vi "Query.vi"(6 "delay (55ms)":u32=55, 8 "error in (no error)":errorcluster, 10 "data in":string, 11 "refnum in":refnum<visa-resource-name>) -> (0 "error out":errorcluster, 2 "data out":string, 3 "refnum out":refnum<visa-resource-name>)   [LabVIEW 2020, in "Korad KA3305P.lvlib"]
uses:
  Korad KA3305P.lvlib
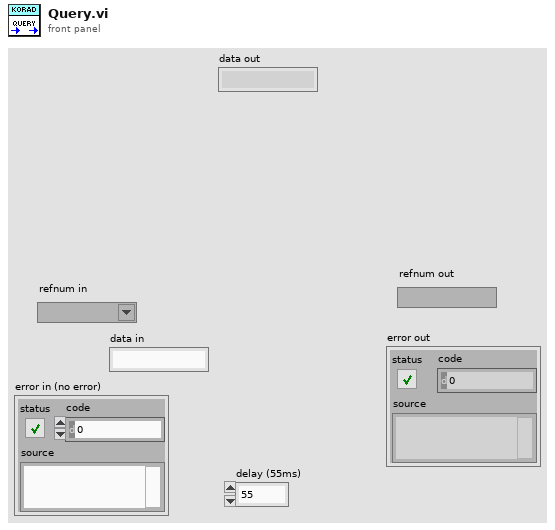
[diagram p1: front panel]
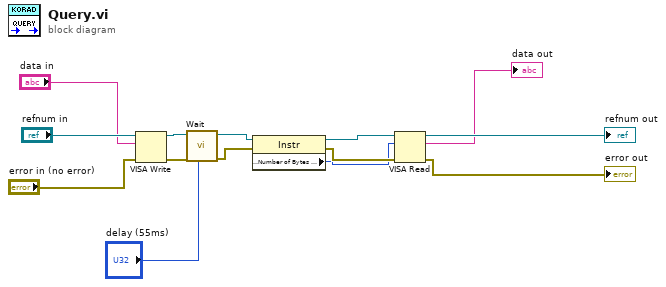
[diagram p0: block diagram]
diagram:
  n1 = VISA Write(VISA resource name="refnum in", write buffer="data in", error in (no error)="error in (no error)") -> (VISA resource name out=w8:refnum<visa-resource-name>, error out=w7:errorcluster)  [unwired: 1 out]
  n2 = call "Wait.vi"("milliseconds to wait"="delay (55ms)", "error in (no error)"=w7, "refnum in"=w8) -> ("error out"=w5:errorcluster, "refnum out"=w6:refnum<visa-resource-name>)  [unwired: 7 in]
  n3 = property class="Instr"(reference=w6, error in=w5) -> (reference out=w2:refnum<visa-resource-name>, error out=w4:errorcluster, "Serial Settings:Number of Bytes at Serial Port"=w3:u32)
  n4 = VISA Read(VISA resource name=w2, byte count=w3, error in (no error)=w4) -> (VISA resource name out=→"refnum out":refnum<visa-resource-name>, read buffer=→"data out":string, error out=→"error out":errorcluster)  [unwired: 1 out]
